vi "BLM_ReadOneDataRegister.vi"(4 "error in (no error)":errorcluster, 5 "Read Echo?":bool, 6 "Register#":string, 7 "Port Address":refnum<visa-resource-name>) -> (0 "error out":errorcluster, 1 "Register Value":dbl, 2 "Register String":string, 3 "Port Address Out":refnum<visa-resource-name>)   [LabVIEW 2025]
doc: "Author: Scott Hannahs <sth@magnet.fsu.edu>\n\nThis software is licensed for use under the “MIT License\"\nCopyright (c) 2025 Scott Hannahs, sth@sth@magnet.sthnet.net\n\nPermission is hereby granted, free of charge, to any person obtaining a copy of this software and associated documentation files (the \"Software\"), to deal in the Software without restriction, including without limitation the rights to use, copy, modify, merge, publish, distribute, sublicense, and/or sell copies of the Software, and to permit persons to whom the Software is furnished to do so, subject to the following conditions: The above copyright notice and this permission notice shall be included in all copies or substantial portions of the Software.\n\nTHE SOFTWARE IS PROVIDED \"AS IS\", WITHOUT WARRANTY OF ANY KIND, EXPRESS OR IMPLIED, INCLUDING BUT NOT LIMITED TO THE WARRANTIES OF MERCHANTABILITY, FITNESS FOR A PARTICULAR PURPOSE AND NONINFRINGEMENT. IN NO EVENT SHALL THE AUTHORS OR COPYRIGHT HOLDERS BE LIABLE FOR ANY CLAIM, DAMAGES OR OTHER LIABILITY, WHETHER IN AN ACTION OF CONTRACT, TORT OR OTHERWISE, ARISING FROM, OUT OF OR IN CONNECTION WITH THE SOFTWARE OR THE USE OR OTHER DEALINGS IN THE SOFTWARE."
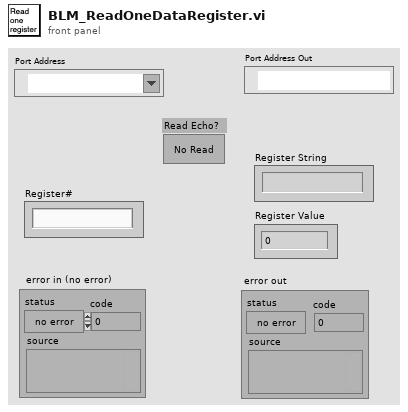
[diagram p1: front panel]
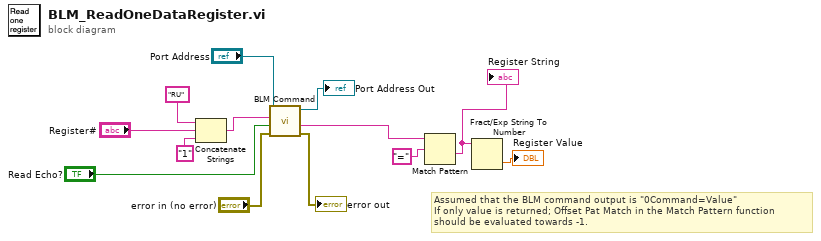
[diagram p0: block diagram]
diagram:
  # "Assumed that the BLM command output is \"0Command=Value\"\nIf only value is returned; Offset Pat Match in the Match Pattern function \nshould be evaluated towards -1."
  n1 = Concatenate Strings("RU" ("Command"), "Register#", "1" ("string")) -> (w2:string)
  n2 = call "BLM Command.vi"("error in (no error)"="error in (no error)", "Read Echo?"="Read Echo?", "Command"=w2, "Port Address"="Port Address") -> ("error out"=→"error out":errorcluster, "Response"=w11:string, "Port Address Out"=→"Port Address Out":refnum<visa-resource-name>)  [unwired: 2 in, 2 out]
  n3 = Match Pattern(string=w11, regular expression="=") -> (after substring=w12:string)  [unwired: 1 in, 3 out]
  "Register String" <- w12
  n4 = Fract/Exp String To Number(string=w12) -> (number=→"Register Value":dbl)  [unwired: 3 in, 1 out]
